vi "GetAttributeViBoolean_SA-Gating_Sweep.vi"(8 "error in (no error)":errorcluster {"code" format="%.0x"}, 9 "AttributeID":u32(ring)=1150527 items=["SA_GATING_ENABLED"=1150527, "SA_GATING_HOLD_OFF_TIME_AUTO_ENABLED"=1150536, "SA_GATING_VIEW"=1150533, "SA_LISTSWEEP_ENABLED"=1150754, "SA_LISTSWEEP_FREQUENCY_SYNTHESIS_AUTO_ENABLED"=1150640, "SA_LISTSWEEP_SEQUENCE_AUTO_ENABLED"=1150642, "SA_SWEEPCOUPLING_BANDWIDTH_RATIO_AUTO_ENABLED"=1150723, "SA_SWEEPCOUPLING_FFT_WIDTH_AUTO_ENABLED"=1150726, "SA_SWEEPCOUPLING_SWEEP_TIME_AUTO_RULES_AUTO_ENABLED"=1150733, "SA_SWEEPCOUPLING_SWEEP_TYPE_AUTO_ENABLED"=1150735, "SA_SWEEPCOUPLING_SWEEP_TYPE_AUTO_RULES_AUTO_ENABLED"=1150729], 11 "instrument handle":refnum<k15>) -> (0 "error out":errorcluster {"code" format="%.0x"}, 2 "AttributeValue":bool, 3 "instrument handle out":refnum<k15>)   [LabVIEW 2009, in "Keysight XSAn.lvlib"]
doc: "Gets a Boolean attribute from the instrument driver.\nThe following Attributes are supported:\n\nSA_GATING_ENABLED\nSA_GATING_HOLD_OFF_TIME_AUTO_ENABLED\nSA_GATING_VIEW\nSA_LISTSWEEP_ENABLED\nSA_LISTSWEEP_FREQUENCY_SYNTHESIS_AUTO_ENABLED\nSA_LISTSWEEP_SEQUENCE_AUTO_ENABLED\nSA_SWEEPCOUPLING_BANDWIDTH_RATIO_AUTO_ENABLED\nSA_SWEEPCOUPLING_FFT_WIDTH_AUTO_ENABLED\nSA_SWEEPCOUPLING_SWEEP_TIME_AUTO_RULES_AUTO_ENABLED\nSA_SWEEPCOUPLING_SWEEP_TYPE_AUTO_ENABLED\nSA_SWEEPCOUPLING_SWEEP_TYPE_AUTO_RULES_AUTO_ENABLED"
uses:
  <instrlib>/Keysight XSAn/Keysight XSAn.lvlib
  AgXSAn.dll
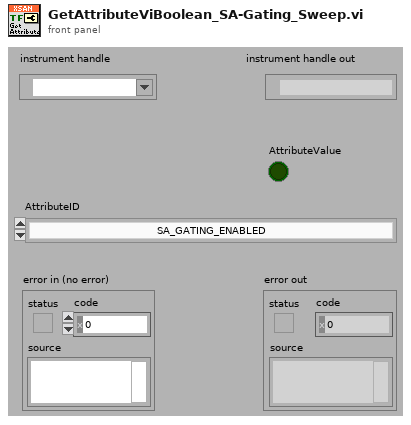
[diagram p1: front panel]
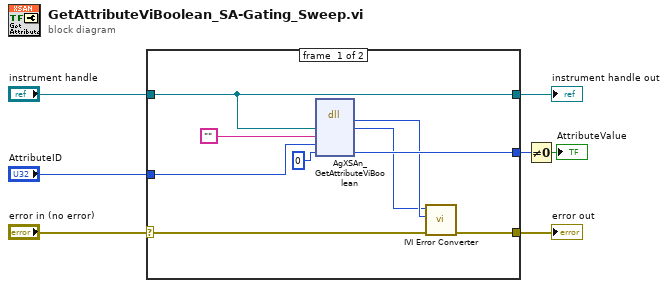
[diagram p0: block diagram]
diagram:
  n1 = case shown="No Error" "error in (no error)" {
    selector: "error in (no error)" -> [w16 w18]
    tunnel: [w15 w18] -> w7
    tunnel: "instrument handle" -> [w11 w17]
    tunnel: "AttributeID" -> [w14 _]
    tunnel: [w12 _] -> w2
    tunnel: [w11 w17] -> w1
    frame #0 {
      n2 = dll-call lib="AgXSAn**.dll" fn="AgXSAn_GetAttributeViBoolean"("Vi"=w11, "RepCapIdentifier"="", "AttributeID"=w14, "AttributeValue"=i16 0) -> ("return type"=w10:i32, "Vi"=w9:u32, "AttributeValue"=w12:i16)  [unwired: 5 in, 2 out]
      n3 = call <instrlib>:"IVI Error Converter.vi"("error in (no error)"=w16, "IVI error code (0)"=w10, "instrument handle"=w9) -> ("error out"=w15:errorcluster)  [unwired: 7 in, 1 out]
    }
    frame #1 {
    }
  }
  "error out" <- w7
  "instrument handle out" <- w1
  n4 = Not Equal To 0?(x=w2) -> (x != 0?=→"AttributeValue":bool)
